vi "niRFUtil MASMT Util Constrained Linear Fit (DBL).vi"(0 "Y":dbl[](array[numeric]), 1 "method":i32(ring) items=["Least Square", "Least Absolute Residual", "Bisquare"], 5 "X":dbl[](array[numeric]), 7 "Weight":dbl[](array[numeric]), 9 "tolerance":dbl=9.999999747378752e-05, 11 "error in (no error)":errorcluster, 12 "parameter bounds":T1={"slope min"=-inf, "slope max"=inf, "intercept min"=-inf, "intercept max"=inf}) -> (4 "Best Linear Fit":dbl[](array[numeric]), 6 "slope":dbl, 8 "intercept":dbl, 10 "residue":dbl, 15 "error out":errorcluster)   [LabVIEW 2015, in "niRFUtil.lvlib"]
uses:
  niRFUtil.lvlib
  <vilib>/Analysis/NI_AALPro.lvlib
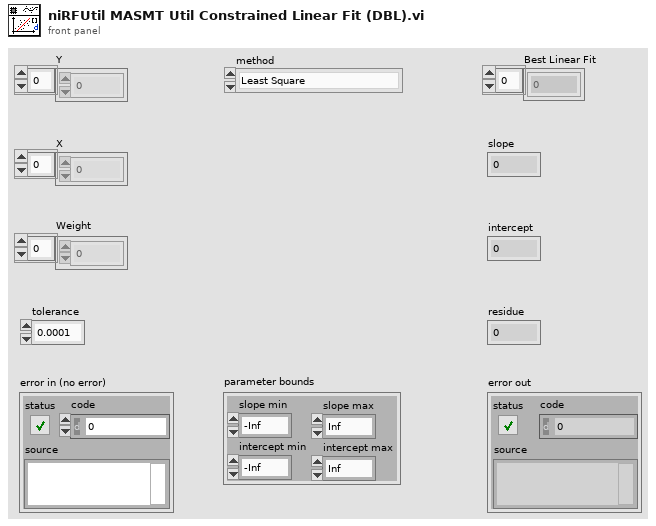
[diagram p1: front panel]
types:
  T1 = cluster{"slope min":dbl, "slope max":dbl, "intercept min":dbl, "intercept max":dbl}
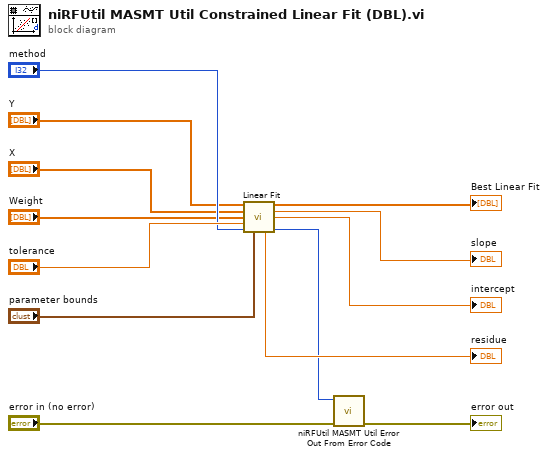
[diagram p0: block diagram]
diagram:
  n1 = call <vilib>:"Linear Fit.vi"("Y"="Y", "X"="X", "Weight"="Weight", "tolerance"="tolerance", "method"="method", "parameter bounds"="parameter bounds") -> ("Best Linear Fit"=→"Best Linear Fit":dbl[], "slope"=→"slope":dbl, "intercept"=→"intercept":dbl, "residue"=→"residue":dbl, "error"=w2:i32)  [unwired: 5 in]
  n2 = call "niRFUtil MASMT Util Error Out From Error Code.vi"("error in (no error)"="error in (no error)", "error code"=w2) -> ("error out"=→"error out":errorcluster)  [unwired: 9 in]
